vi "SetAppStrConstant--function.vi"(8 "error in":errorcluster, 9 "Value":string, 10 "Label.Text":string, 11 "vi path":path) -> (0 "error out":errorcluster, 2 "found?":bool)   [LabVIEW 2020, in "CICD.lvlib"]
doc: "Sets the value in a string constant programmatically.\nCall this VI from LabVIEWCLI or GCLI to update a LabVIEW constant (e.g. app version) before building from the CI server."
uses:
  CICD.lvlib
  <vilib>/Utility/error.llb/Error Cluster From Error Code.vi
  <vilib>/ErrorRing/Error Ring.xnode
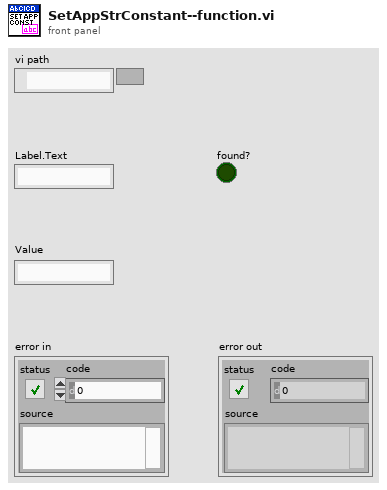
[diagram p1: front panel]
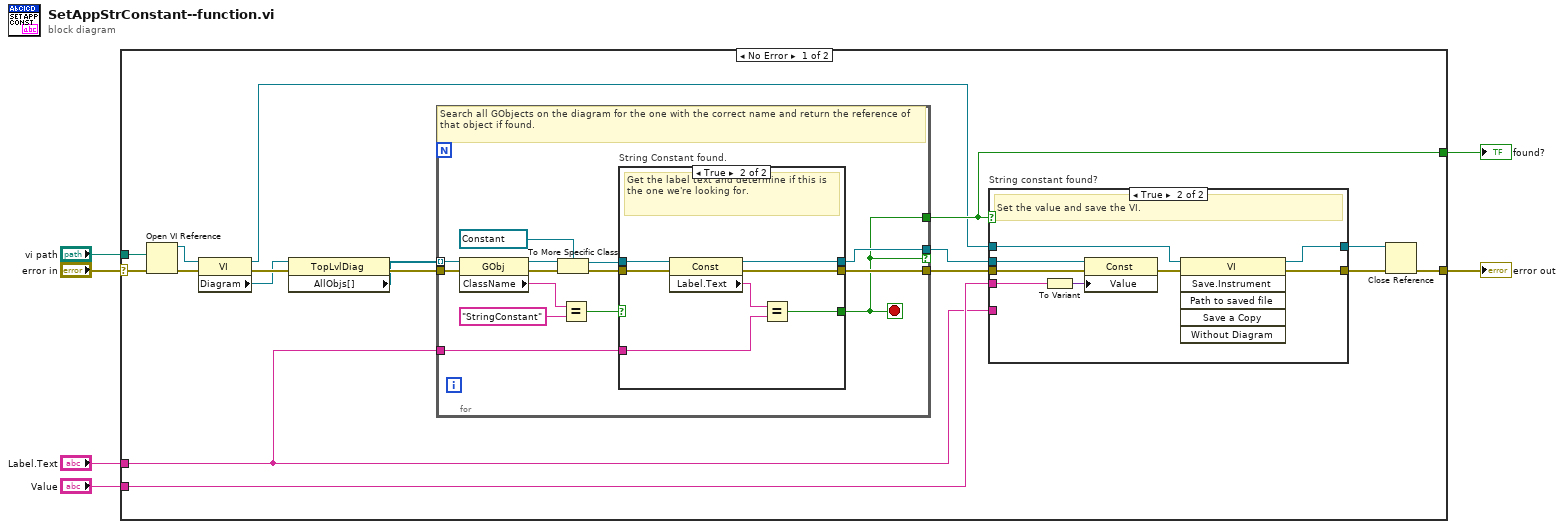
[diagram p0: block diagram]
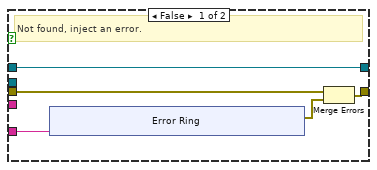
[diagram p2: hidden frame]
diagram:
  n1 = case shown="No Error" "error in" {
    selector: "error in" -> [w7 w67]
    tunnel: [w20 w67] -> w6
    tunnel: "Value" -> [w16 _]
    tunnel: "vi path" -> [w13 _]
    tunnel: [w11 _] -> w3
    tunnel: "Label.Text" -> [w10 _]
    frame No Error {
      n2 = Open VI Reference(vi path=w13, error in (no error)=w7) -> (vi reference=w14:refnum<vi>, error out=w21:errorcluster)  [unwired: 4 in]
      n3 = property on="Property Node" class="VI"(reference=w14, error in=w21) -> (reference out=w8:refnum<vi>, error out=w23:errorcluster, "Diagram"=w15:refnum<vi>)
      n4 = property on="Property Node" class="TopLvlDiag"(reference=w15, error in=w23) -> (error out=w22:errorcluster, "AllObjs[]"=w17:refnum<vi>[])  [unwired: 1 out]
      n5 = for {
        tunnel: w17 -> [w53] mode=indexing
        tunnel: w22 -> [w57]
        tunnel: w10 -> [w50]
        tunnel: [w49] -> w12 if=w47
        tunnel: [w55] -> w19
        tunnel: [w47] -> w11
        stop <- w47 stop-if-true
        # "Search all GObjects on the diagram for the one with the correct name and return the reference of that object if found."
        n6 = property class="GObj"(reference=w53, error in=w57) -> (reference out=w46:refnum<vi>, error out=w56:errorcluster, "ClassName"=w52:string)
        n7 = To More Specific Class(target class=refnum<vi> refnum ("reference"), reference=w46, error in=w56) -> (specific class reference=w45:refnum<vi>, error out=w54:errorcluster)
        n8 = Equal?(x=w52, y="StringConstant" ("x")) -> (x = y?=w48:bool)
        n9 = case "String Constant found." shown="True" w48 {
          tunnel: w54 -> [w59 w66]
          tunnel: w45 -> [w58 w64]
          tunnel: w50 -> [_ w62]
          tunnel: [w58 w61] -> w49
          tunnel: [_ w60] -> w47
          tunnel: [w59 w65] -> w55
          frame False {
            # "Not found, continue."
          }
          frame True {
            # "Get the label text and determine if this is the one we're looking for."
            n10 = property on="Property Node" class="Const"(reference=w64, error in=w66) -> (reference out=w61:refnum<vi>, error out=w65:errorcluster, "Label.Text"=w63:string)
            n11 = Equal?(x=w63, y=w62) -> (x = y?=w60:bool)
          }
        }
      }
      n12 = case "String constant found?" shown="True" w11 {
        tunnel: w16 -> [_ w39]
        tunnel: w19 -> [w27 w43]
        tunnel: w12 -> [_ w38]
        tunnel: [w28 w41] -> w18
        tunnel: w10 -> [w25 _]
        tunnel: [w24 w37] -> w9
        tunnel: w8 -> [w24 w36]
        frame False {
          # "Not found, inject an error."
          n13 = xnode "Error Ring"("parameter 0"=w25) -> ("error out"=w26:errorcluster)
          n14 = Merge Errors(w27, w26) -> (w28:errorcluster)
        }
        frame True {
          # "Set the value and save the VI."
          n15 = To Variant(anything=w39) -> (Variant=w40:variant)
          n16 = property on="Property Node" class="Const"(reference=w38, error in=w43, "Value"=w40) -> (error out=w42:errorcluster)  [unwired: 1 out]
          n17 = invoke class="VI" method="Save.Instrument"(reference=w36, error in=w42) -> (reference out=w37:refnum<vi>, error out=w41:errorcluster)  [unwired: 4 in, 4 out]
        }
      }
      n18 = Close Reference(reference=w9, error in (no error)=w18) -> (error out=w20:errorcluster)
    }
    frame Error {
    }
  }
  "error out" <- w6
  "found?" <- w3
